vi "Add Menu Items.vi"(0 "Display State In":T1, 5 "Menu":string[](array[string]), 7 "index":i32, 9 "Container State":T4, 11 "error in (no error)":errorcluster) -> (4 "Display State Out":T1, 15 "error out":errorcluster)   [LabVIEW 2013, in "UI Panels.lvlib" / "Panels_XControl.xctl"]
uses:
  Panels_XControl.xctl
  <vilib>/_xctls/Container State.ctl
  State 1.ctl
  Controls/References/Panel_Refnums.ctl
  Controls/Panel_Command_Enum.ctl
  <vilib>/_xctls/XControlSupport.lvlib
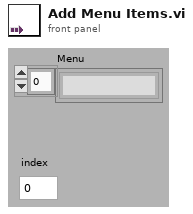
[diagram p1: front panel]
types:
  T1 = typedef "UI Panels.lvlib/Panels_XControl.xctl/State 1.ctl" = cluster{"Panels_Refnums_Array":T2[], "Panel_Command":cluster{"Operation":T3, "Data":variant}}
  T2 = typedef "UI Panels.lvlib/Panels_XControl.xctl/Panel_Refnums.ctl" = cluster{"VI Refnum":refnum<vi>, "Command":refnum<user-event>, "Visible":bool}
  T3 = typedef "UI Panels.lvlib/Panels_XControl.xctl/Panel_Command_Enum.ctl" = enum16{"Idle", "Remove & Stop", "Add Item", "Delete Item", "Delete All", "Insert into Subpanel", "Register Menu Events", "Update Value", "Remove from Subpanel", "Set Title", "Set Menu Items", "Insert SubPanel", "Set Splitter Position", "Set Splitter Properties", "Add Menu Items"}
  T4 = typedef "XControlSupport.lvlib/Container State.ctl" = cluster{"Indicator?":bool, "Run Mode?":bool, " Refnum":refnum<vi>}
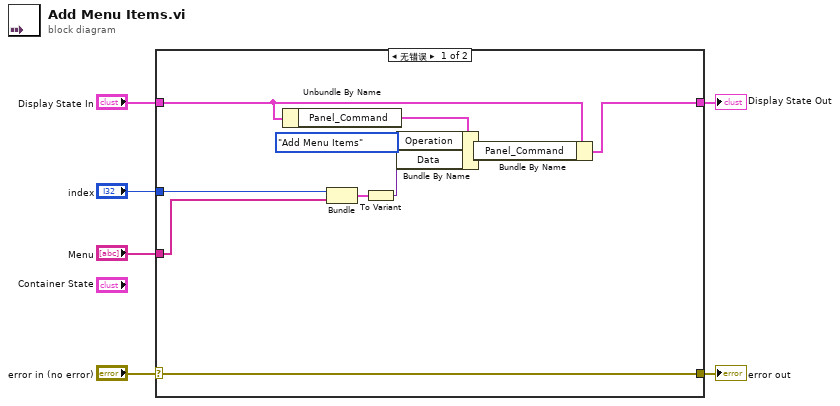
[diagram p0: block diagram]
diagram:
  n1 = case shown="无错误" "error in (no error)" {
    selector: "error in (no error)" -> [w8 w18]
    tunnel: "index" -> [w12 _]
    tunnel: [w10 w17] -> w5
    tunnel: "Display State In" -> [w9 w17]
    tunnel: "Menu" -> [w7 _]
    tunnel: [w8 w18] -> w2
    frame No Error {
      n2 = Unbundle By Name(w9) -> ("Panel_Command"=w13:cluster{"Operation":T3, "Data":variant})
      n3 = Bundle("index"=w12, "Menu"=w7) -> (w11:cluster{"index":i32, "Menu":string[]})  [unwired: 1 out]
      n4 = To Variant(anything=w11) -> (Variant=w15:variant)
      n5 = Bundle By Name(cluster=w13, "Operation"=Panel_Command_Enum."Add Menu Items", "Data"=w15) -> (w16:cluster{"Operation":T3, "Data":variant})
      n6 = Bundle By Name(cluster=w9, "Panel_Command"=w16) -> (w10:T1)
    }
    frame Error {
    }
  }
  "Display State Out" <- w5
  "error out" <- w2
